vi "Write Initial Values.vi"(8 "error in (no error)":errorcluster, 10 "Initial Values":refnum<class "Abs_Value.lvclass">[](array[class]), 11 "Local Bus in":refnum<class "Local Bus.lvclass">) -> (0 "error out":errorcluster, 3 "Local Bus out":refnum<class "Local Bus.lvclass">)   [LabVIEW 2021, in "Local Bus.lvclass"]
uses:
  Local Bus.lvclass
  Local Bus.lvclass/Local Bus.ctl
  <vilib>/TSA/Abstract Data Classes/Abs_Types/Value/Abs_Value.lvclass
  C:/Program Files (x86)/National Instruments/LabVIEW 2021/vi.lib/TSA/Abstract Data Classes/Abs_Types/Type/Abs_Type.lvclass
  C:/Program Files (x86)/National Instruments/LabVIEW 2021/vi.lib/TSA/Abstract Data Classes/Abs_Types/Value/Abs_Value.lvclass
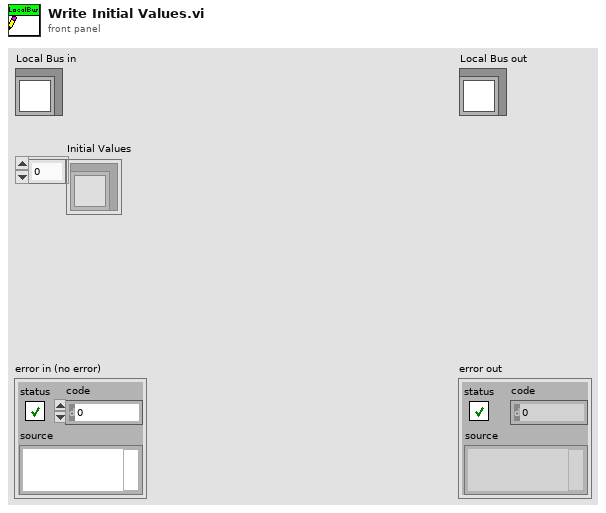
[diagram p1: front panel]
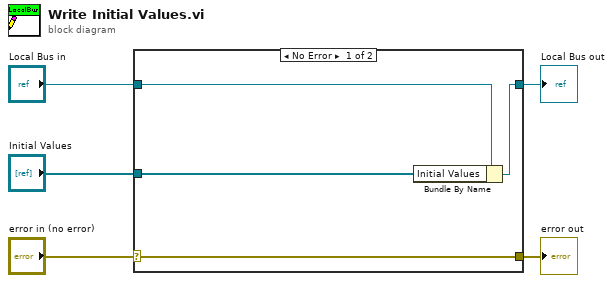
[diagram p0: block diagram]
diagram:
  n1 = case shown="No Error" "error in (no error)" {
    selector: "error in (no error)" -> [w9 w10]
    tunnel: [w9 w10] -> w4
    tunnel: [w7 w11] -> w2
    tunnel: "Local Bus in" -> [w8 w11]
    tunnel: "Initial Values" -> [w6 _]
    frame No Error {
      n2 = Bundle By Name(cluster=w8, "Initial Values"=w6) -> (w7:refnum<class "Local Bus.lvclass">)
    }
    frame Error {
    }
  }
  "error out" <- w4
  "Local Bus out" <- w2
